vi "as_global.vi"() -> ()   [LabVIEW 2013]
panel:
  out "Parameter List Path":path
  out "Stimulus List Path":path
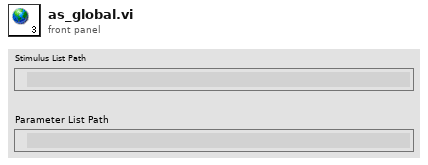
[diagram p1: front panel]
diagram:
